vi "Select Request Objects.vi"(11 "Processing In":refnum<class "Processing.lvclass">) -> (3 "Processing":refnum<class "Processing.lvclass">, 5 "Early Response?":bool, 7 "Trace Message":string)   [LabVIEW 2020, in "HTTP Server.lvlib" / "Server.lvclass"]
uses:
  Server.lvclass
  lv-http-util/HTTP Utils/Response/Response.lvclass
  Processing/Processing.lvclass
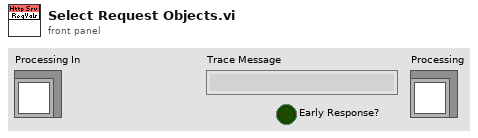
[diagram p1: front panel]
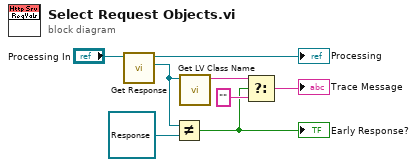
[diagram p0: block diagram]
diagram:
  n1 = call "Get Response.vi"("Processing in"="Processing In") -> ("Response"=w2:refnum<class "Response.lvclass">, "Processing out"=→"Processing":refnum<class "Processing.lvclass">)  [unwired: 9 in]
  n2 = Not Equal?(x=w2, y=refnum<class "Response.lvclass"> refnum) -> (x != y?=w5:bool)
  "Early Response?" <- w5
  n3 = call <vilib>:"Get LV Class Name.vi"("object"=w2) -> ("class name"=w7:string)  [unwired: 9 in, 1 out]
  n4 = Select(t=w7, s=w5, f="") -> (s? t:f=→"Trace Message":string)
